vi "Get Setpoints.vi"(0 "object in":refnum<class "HPS-17000-PowerModule.lvclass">, 11 "Error In":errorcluster) -> (4 "object out":refnum<class "HPS-17000-PowerModule.lvclass">, 6 "current (A)":dbl, 8 "voltage (V)":dbl, 10 "resistance (Ohms)":dbl, 15 "Error Out":errorcluster)   [LabVIEW 2023, in "HPS-17000-PowerModule.lvlib" / "HPS-17000-PowerModule.lvclass"]
uses:
  HPS-17000-PowerModule.lvclass
  <vilib>/Utility/error.llb/Trim Whitespace One-Sided.vi
  HPS-17000-PowerModule.lvclass/HPS-17000-PowerModule.ctl
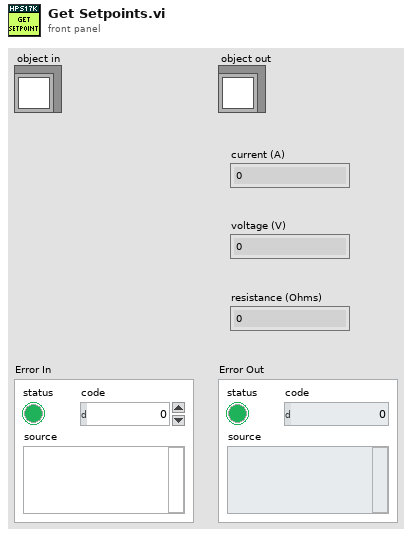
[diagram p1: front panel]
types:
  T1 = typedef "HPS-17000-PowerModule.lvlib/HPS-17000-PowerModule.lvclass/ObjectAttributes.ctl" = cluster{"Configuration":cluster{"TSN NIC IP Address":string, "HPS17000 IP Addresses":string[], "HPS Topology":enum16{"SINGLE", "MULTI"}, "Setpoint Stream Config":T2, "Limits":T3}, "GM ID":string, "HPS17000 Refs":refnum<class "HPS-17000.lvclass">[], "Stream Queues":refnum<queue>[], "connected":bool, "reserved":bool, "events":T4, "nibatterycycler_grpc_Setpoint":T5, "last timestamp":i64, "mode":T6, "range":T7}
  T2 = typedef "Cycler.lvclass/Setpoint Stream Basic Config.ctl" = cluster{"local address":string, "receiver port":u16}
  T3 = typedef "PowerModuleInterface.lvlibp/PowerModuleInterface.lvclass/Limits.ctl" = cluster{"Current Max (A)":dbl, "Current Min (A)":dbl, "Voltage Max (V)":dbl, "Voltage Min (V)":dbl, "Power Max (W)":dbl, "Power Min (W)":dbl}
  T4 = typedef "HPS-17000.lvclass/Multi-Cycler Events.ctl" = cluster{"heartbeats events":refnum<user-event>[], "faults events":refnum<user-event>[], "network sync event":refnum<user-event>[], "setpoint status event":refnum<user-event>[]}
  T5 = typedef "NI_BC_client.lvlib/nibatterycycler_grpc_Setpoint.ctl" = cluster{"voltage":sgl, "current":sgl, "min_power":sgl, "max_power":sgl, "resistance":sgl}
  T6 = typedef "HPS-17000-PowerModule.lvlib/HPS-17000-PowerModule.lvclass/Mode.ctl" = u16
  T7 = typedef "PowerModuleInterface.lvlibp/PowerModuleInterface.lvclass/Range.ctl" = cluster{"Current Max (A)":dbl, "Current Min (A)":dbl, "Voltage Max (V)":dbl, "Voltage Min (V)":dbl}
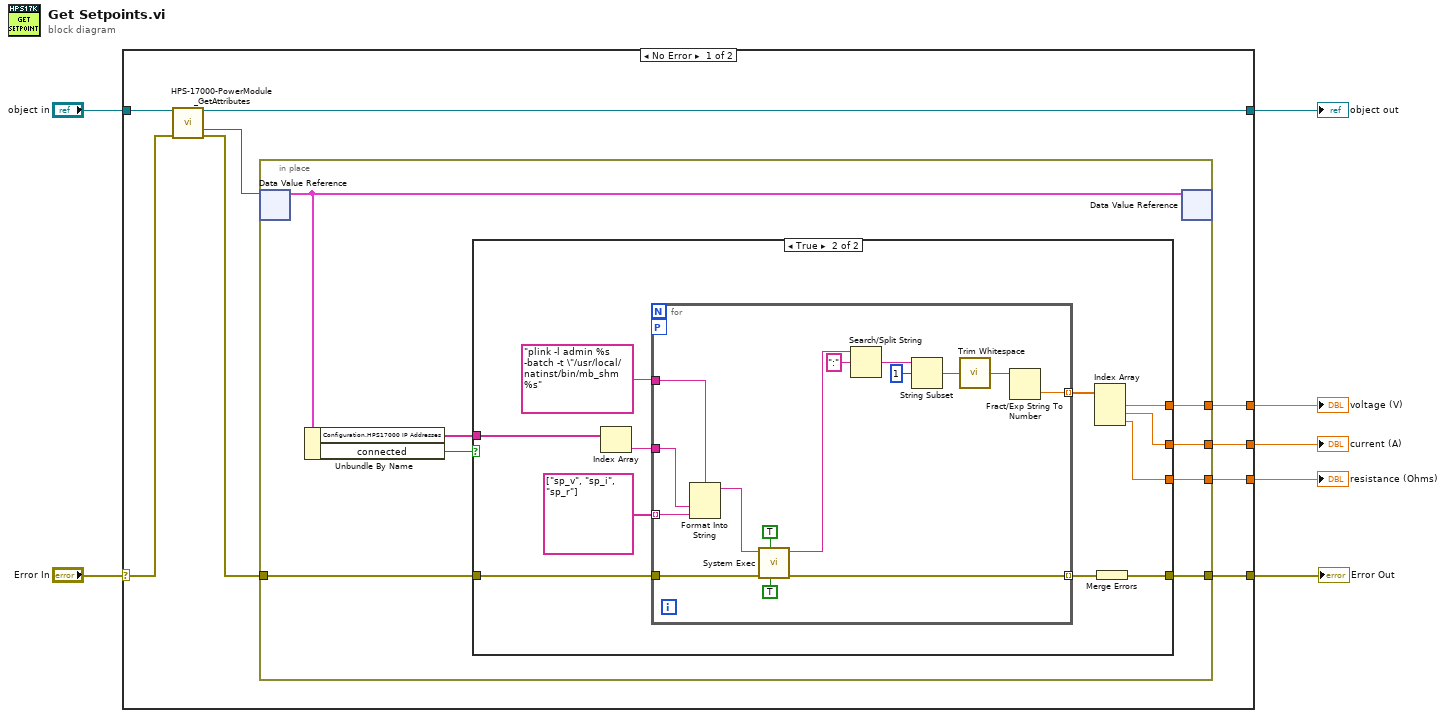
[diagram p0: block diagram]
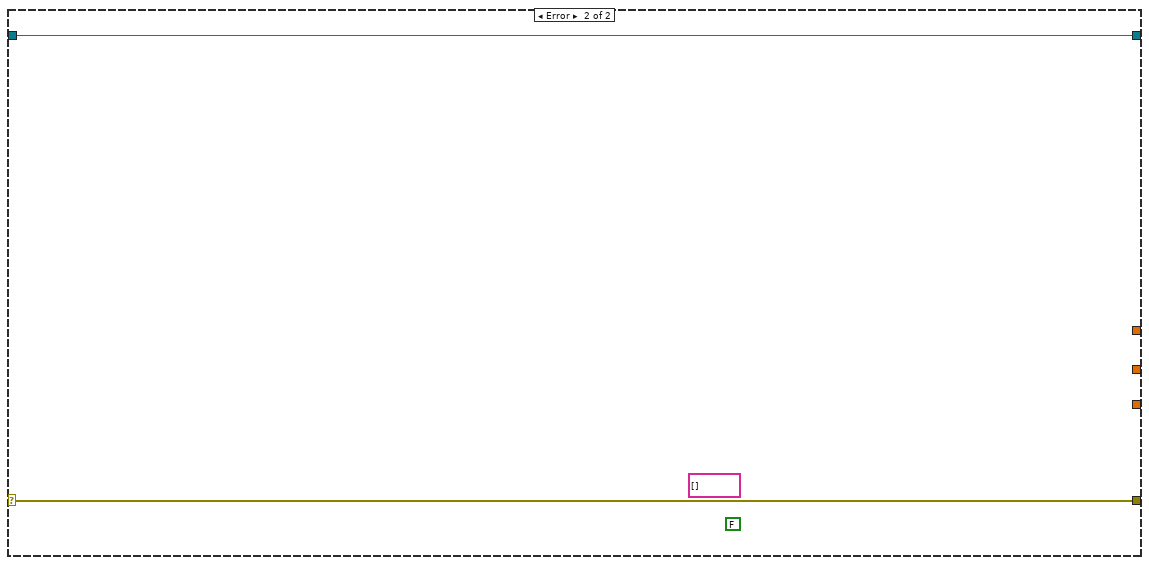
[diagram p3: hidden frame]
diagram:
  n1 = case shown="No Error" "Error In" {
    selector: "Error In" -> [w15 w52]
    tunnel: "object in" -> [w16 w53]
    tunnel: [w11 w53] -> w6
    tunnel: [w12 w52] -> w4
    tunnel: [w10 _] -> w3
    tunnel: [w9 _] -> w2
    tunnel: [w8 _] -> w1
    frame No Error {
      n2 = call "HPS-17000-PowerModule_GetAttributes.vi"("reference in"=w16, "Error In"=w15) -> ("reference out"=w11:refnum<class "HPS-17000-PowerModule.lvclass">, "DataRef"=w14:refnum<data-value>, "Error Out"=w13:errorcluster)  [unwired: 10 in, 1 out]
      n3 = in-place {
        in-place-border: w13 -> [w24]
        in-place-border: [w23] -> w12
        in-place-border: [w19] -> w10
        in-place-border: [w18] -> w9
        in-place-border: [w17] -> w8
        n4 = in-place-dvr #1(w14) -> (w21:T1)  [unwired: 1 out]
        n5 = Unbundle By Name(w21) -> ("Configuration.HPS17000 IP Addresses"=w20:string[], "connected"=w22:bool)
        n6 = case shown="True" w22 {
          tunnel: w24 -> [w25 w34]
          tunnel: [w25 w32] -> w23
          tunnel: w20 -> [_ w31]
          tunnel: [_ w28] -> w19
          tunnel: [_ w27] -> w18
          tunnel: [_ w26] -> w17
          frame False {
          }
          frame True {
            n7 = Index Array(array=w31) -> (element=w30:string)  [unwired: 1 in]
            n8 = for {
              tunnel: w34 -> [w49]
              tunnel: [w44] -> w33 mode=indexing
              tunnel: "plink -l admin %s -batch -t \"/usr/local/natinst/bin/mb_shm %s" ("format string") -> [w48]
              tunnel: string[] ["sp_v", "sp_i", "sp_r"] -> [w46] mode=indexing
              workers-P: _ -> [_]
              tunnel: [w42] -> w29 mode=indexing
              tunnel: w30 -> [w37]
              n9 = Format Into String(format string=w48, w37, w46) -> (resulting string=w47:string)  [unwired: 2 in, 1 out]
              n10 = call <vilib>:"System Exec.vi"("run minimized? (F)"=TRUE, "wait until completion? (T)"=TRUE, "error in (no error)"=w49, "command line"=w47) -> ("error out"=w44:errorcluster, "standard output"=w41:string)  [unwired: 4 in, 2 out]
              n11 = Search/Split String(string=w41, search string/char (-)=":") -> (match + rest of string=w39:string)  [unwired: 1 in, 2 out]
              n12 = String Subset(string=w39, offset (0)=1) -> (substring=w38:string)  [unwired: 1 in]
              n13 = call <vilib>:"Trim Whitespace.vi"("string"=w38) -> ("trimmed string"=w43:string)  [unwired: 1 in]
              n14 = Fract/Exp String To Number(string=w43) -> (number=w42:dbl)  [unwired: 3 in, 1 out]
            }
            n15 = Index Array(array=w29) -> (element #1=w28:dbl, element #2=w27:dbl, element #3=w26:dbl)  [unwired: 3 in]
            n16 = Merge Errors(w33) -> (w32:errorcluster)
          }
        }
        n17 = in-place-dvr #1(w21) -> ()  [unwired: 2 out]
      }
    }
    frame Error {
      (unwired) string[] []
      (unwired) FALSE
    }
  }
  "Error Out" <- w4
  "object out" <- w6
  "current (A)" <- w2
  "voltage (V)" <- w3
  "resistance (Ohms)" <- w1
